vi "Init.vi"(8 "error in (no error)":errorcluster, 11 "Report In":refnum<class "Report.lvclass">) -> (0 "error out":errorcluster, 3 "Report Out":refnum<class "Report.lvclass">)   [LabVIEW 2020, in "Reports.lvlib" / "Report.lvclass"]
uses:
  Report.lvclass
  C:/git/astemes-lunit/source/Framework/Report Interface/Report Interface.lvclass
  Report.lvclass/Report.ctl
  Report Generator/Report Generator.lvclass
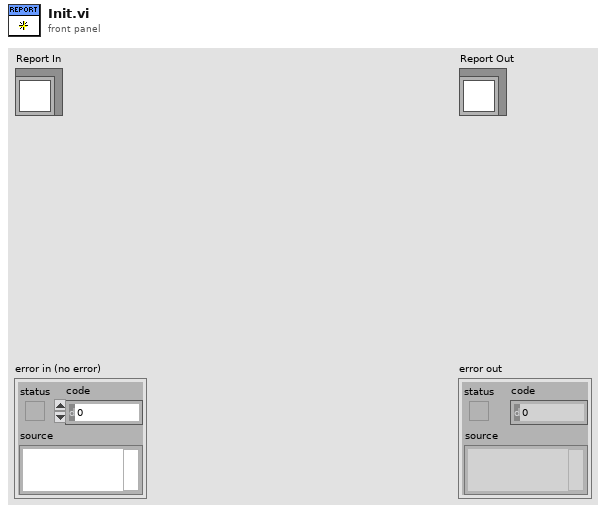
[diagram p1: front panel]
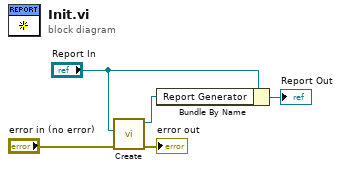
[diagram p0: block diagram]
diagram:
  n1 = call "Create.vi"("error in (no error)"="error in (no error)", "Report"="Report In") -> ("error out"=→"error out":errorcluster, "Report Generator Out"=w2:refnum<class "Report Generator.lvclass">)  [unwired: 8 in]
  n2 = Bundle By Name(cluster="Report In", "Report Generator"=w2) -> (→"Report Out":refnum<class "Report.lvclass">)
